vi "pb_get_firmware.vi"(8 "error in (no error)":errorcluster, 11 "path in":path) -> (0 "error out":errorcluster, 3 "path out":path)   [LabVIEW 2016]
panel:
  out "return type":i32
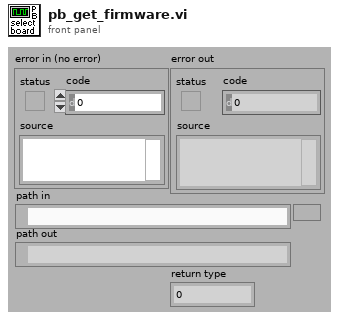
[diagram p1: front panel]
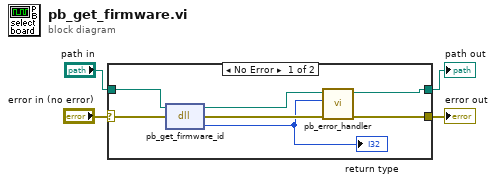
[diagram p0: block diagram]
diagram:
  n1 = case shown="No Error" "error in (no error)" {
    selector: "error in (no error)" -> [w11 w13]
    tunnel: [w6 w13] -> w3
    tunnel: "path in" -> [w10 w12]
    tunnel: [w8 w12] -> w1
    frame No Error {
      n2 = dll-call lib="C:/Program Files/SpinCore/SpinAPI/dll/spinapi.dll" fn="pb_get_firmware_id"(path in=w10, error in=w11) -> (path out=w9:path, error out=w7:errorcluster, "return type"=w5:i32)  [unwired: 1 in]
      "return type" <- w5
      n3 = call "pb_error_handler.vi"("error in (no error)"=w7, "return code"=w5, "path in"=w9) -> ("error out"=w6:errorcluster, "path out"=w8:path)  [unwired: 7 out]
    }
    frame Error {
    }
  }
  "error out" <- w3
  "path out" <- w1
